vi "Set Config.vi"(5 "Copy Data? [T]":bool=TRUE, 7 "Copy Paths? [T]":bool=TRUE, 8 "error in (no error)":errorcluster, 10 "Carya Config source":refnum<class "Carya Config.lvclass">, 11 "Carya Config dest":refnum<class "Carya Config.lvclass">) -> (0 "error out":errorcluster, 3 "Carya Config out":refnum<class "Carya Config.lvclass">)   [LabVIEW 2013, in "Carya Config.lvclass"]
doc: "Copyright 2018, Carya Automatisering, Wiebe Walstra."
uses:
  Carya Config.lvclass
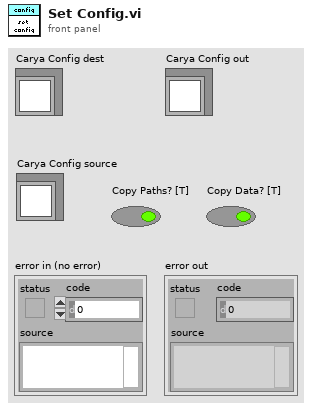
[diagram p1: front panel]
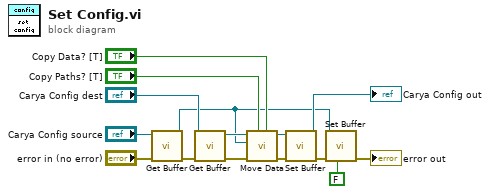
[diagram p0: block diagram]
diagram:
  n1 = call-dynamic "Get Buffer.vi"("error in (no error)"="error in (no error)", "Carya Config in"="Carya Config source") -> ("error out"=w6:errorcluster, "Config"=w2:refnum<class "Carya Config.lvclass">)  [unwired: 8 in]
  n2 = call-dynamic "Get Buffer.vi"("error in (no error)"=w6, "Carya Config in"="Carya Config dest") -> ("error out"=w13:errorcluster, "Config"=w14:refnum<class "Carya Config.lvclass">)  [unwired: 8 in]
  n3 = call "Move Data.vi"("Copy Data? [T]"="Copy Data? [T]", "Copy Paths? [T]"="Copy Paths? [T]", "error in (no error)"=w13, "Carya Config source"=w2, "Carya Config dest"=w14) -> ("error out"=w10:errorcluster, "Carya Config out"=w12:refnum<class "Carya Config.lvclass">)  [unwired: 5 in]
  n4 = call-dynamic "Set Buffer.vi"("error in (no error)"=w10, "Carya Config"=w12) -> ("error out"=w4:errorcluster, "Carya Config out"=→"Carya Config out":refnum<class "Carya Config.lvclass">)  [unwired: 8 in]
  n5 = call-dynamic "Set Buffer.vi"("Set? [T]"=FALSE, "error in (no error)"=w4, "Carya Config"=w2) -> ("error out"=→"error out":errorcluster)  [unwired: 7 in, 1 out]
